vi "ray_direction.vi"(3 "Axis positions":dbl[][](array[numeric]) format="%#_6f", 4 "first axis":i32, 5 "K":T1, 6 "T":T1) -> (1 "Ray directions":T1)   [LabVIEW 2011]
uses:
  <vilib>/Analysis/Matrix/Datatypes/RealMatrix.ctl
  <vilib>/Analysis/Matrix/Numeric/Conversions/Array To Matrix - RA.vi
  <vilib>/Analysis/baseanly.llb/Real A x B.vi
  utilities/labview/norm_mat.vi
  <vilib>/Analysis/Matrix/NI_Matrix.lvlib
  <vilib>/Analysis/NI_AALBase.lvlib
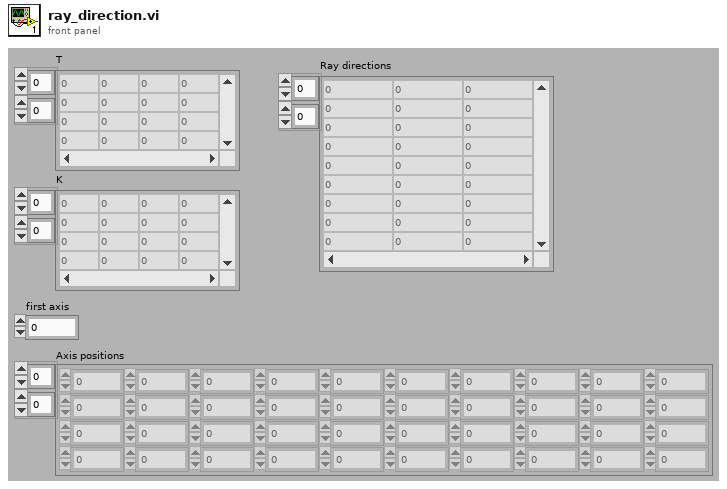
[diagram p1: front panel]
types:
  T1 = typedef "NI_Matrix.lvlib/RealMatrix.ctl" = dbl[][]
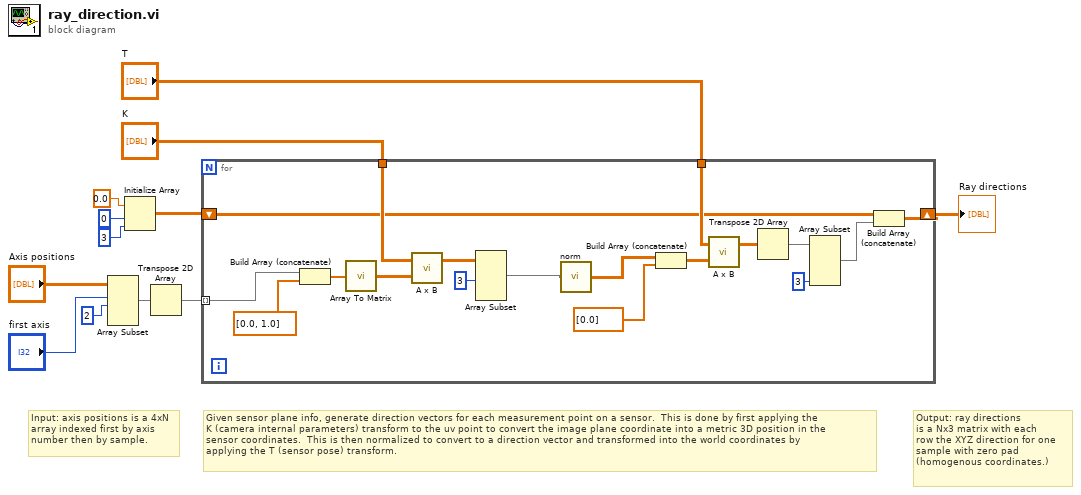
[diagram p0: block diagram]
diagram:
  # "Output: ray directions\nis a Nx3 matrix with each\nrow the XYZ direction for one\nsample with zero pad\n(homogenous coordinates.)"
  # "Input: axis positions is a 4xN\narray indexed first by axis\nnumber then by sample."
  # "Given sensor plane info, generate direction vectors for each measurement point on a sensor.  This is done by first applying the\nK (camera internal parameters) transform to the uv point to convert the image plane coordinate into a metric 3D position in the\nsensor coordinates.  This is then normalized to convert to a direction vector and transformed into the world coordinates by\napplying the T (sensor pose) transform."
  n1 = Array Subset(array="Axis positions", index (row)="first axis", length (row)=2 ("length")) -> (w9:dbl[][])  [unwired: 2 in]
  n2 = Initialize Array(0.0 ("element"), 0 ("dimension size"), 3 ("dimension size")) -> (w3:dbl[][])
  n3 = Transpose 2D Array(2D array=w9) -> (transposed array=w10:dbl[][])
  n4 = for {
    tunnel: w10 -> [w30] mode=indexing
    tunnel: "K" -> [w27]
    tunnel: "T" -> [w22]
    shift-right: [w18] -> w1
    shift-left: w3 -> [w19]
    n5 = Build Array (concatenate)(w30, dbl[] [0.0, 1.0] ("element")) -> (w28:dbl[])
    n6 = call-poly <vilib>:"Array To Matrix.vi"("Real 1D Array"=w28) -> ("Real Matrix (Column Vector)"=w26:T1)
    n7 = call-poly <vilib>:"A x B.vi"("B"=w26, "A"=w27) -> ("A x B"=w25:T1)  [unwired: 1 out]
    n8 = Array Subset(array=w25, length (row)=3 ("length")) -> (w14:T1)  [unwired: 3 in]
    n9 = call-poly "norm.vi"("vector"=w14) -> ("normalized vector"=w13:T1)  [unwired: 4 out]
    n10 = Build Array (concatenate)(w13, dbl[] [0.0] ("element")) -> (w21:T1)
    n11 = call-poly <vilib>:"A x B.vi"("B"=w21, "A"=w22) -> ("A x B"=w20:T1)  [unwired: 1 out]
    n12 = Transpose 2D Array(2D array=w20) -> (transposed array=w17:T1)
    n13 = Array Subset(array=w17, length (col)=3 ("length")) -> (w15:T1)  [unwired: 3 in]
    n14 = Build Array (concatenate)(w19, w15) -> (w18:T1)
  }
  "Ray directions" <- w1
